vi "Create AFDX IP (Dest).vi"(11 "VL":u16) -> (2 "ip string":string, 3 "ip net":u32)   [LabVIEW 2020, in "EthFrameManagement.lvlib"]
uses:
  EthFrameManagement.lvlib
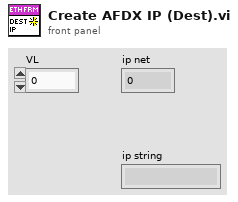
[diagram p1: front panel]
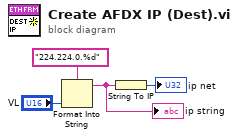
[diagram p0: block diagram]
diagram:
  n1 = Format Into String(format string="224.224.0.%d", "VL") -> (resulting string=w1:string)  [unwired: 2 in, 1 out]
  "ip string" <- w1
  n2 = String To IP(1:w1) -> (0:→"ip net":u32)
